vi "dfd_Validate Multirate Filter.vi"(8 "error in (no error)":errorcluster, 9 "skip FXP? (T)":bool=TRUE, 10 "preferred structure":enum16{"CIC", "FIR", "IIR", "Lattice"}(ring), 11 "multirate filter in":T1={"mMRate_Structure"=enum."CIC", "mMRate_Mode"=0, "mMRate_Factor"=1, "mMRate_FIRParams"={"mMRate_FIR_H"=[], "mMRate_FIR_IsNyquist?"=FALSE, "mMRate_FIR_IsSymmetric?"=FALSE}, "mMRate_CICParams"={"mMRate_CIC_#Stage"=2, "mMRate_CIC_Lag"=1, "mMRate_CIC_Type"=enum."Lowpass"}, "mMRate_Order"=1, "mMRate_Version"="1.0", "mMRate_Comments"="1.0", "mMRate_RationalFactor"={"mMRate_L"=-1, "mMRate_M"=-1}, "mMRate_Fs"=0.0, "mMRate_Quantized?"=FALSE, "mMRate_QFilterGain"=1.0, "mMRate_CoefWl"=16, "mMRate_Scaling"={"mMRate_ScaleByPowerOf2?"=FALSE, "mMRate_ScaleType"=enum."Time Domain 1-Norm"}, "mMRate_InputWl"=0, "mMRate_OutputWl"=0, "mMRate_OutputMode"=enum."Nearest", "mMRate_MultMode"=enum."Full", "mMRate_BitPruning"=FALSE, "mMRate_GainWl"=16, "mMRate_OutputFwl"=0, "mMRate_SumIwl"=0, "mMRate_InputIwl "=16, "mMRate_SumWl"=32, "mMRate_CoefIwl"=0} {"mMRate_SumWl" min=1 max=32 step=1; "mMRate_InputIwl" min=1 max=32 step=1; "mMRate_GainWl" min=1 max=32 step=1; "mMRate_OutputWl" min=1 max=32 step=1; "mMRate_InputWl" min=1 max=32 step=1; "mMRate_CoefWl" min=1 max=32 step=1; "mMRate_Mode" items=["Default"=-1, "No Rate Change"=0, "Interpolation"=1, "Decimation"=2, "Interpolated"=3, "Rational"=4]}) -> (0 "error out":errorcluster, 1 "is Valid FXP?":bool, 2 "is Valid FLP?":bool, 3 "multirate filter out":T1={"mMRate_Structure"=enum."CIC", "mMRate_Mode"=0, "mMRate_Factor"=1, "mMRate_FIRParams"={"mMRate_FIR_H"=[], "mMRate_FIR_IsNyquist?"=FALSE, "mMRate_FIR_IsSymmetric?"=FALSE}, "mMRate_CICParams"={"mMRate_CIC_#Stage"=2, "mMRate_CIC_Lag"=1, "mMRate_CIC_Type"=enum."Lowpass"}, "mMRate_Order"=1, "mMRate_Version"="1.0", "mMRate_Comments"="1.0", "mMRate_RationalFactor"={"mMRate_L"=-1, "mMRate_M"=-1}, "mMRate_Fs"=0.0, "mMRate_Quantized?"=FALSE, "mMRate_QFilterGain"=1.0, "mMRate_CoefWl"=16, "mMRate_Scaling"={"mMRate_ScaleByPowerOf2?"=FALSE, "mMRate_ScaleType"=enum."Time Domain 1-Norm"}, "mMRate_InputWl"=0, "mMRate_OutputWl"=0, "mMRate_OutputMode"=enum."Nearest", "mMRate_MultMode"=enum."Full", "mMRate_BitPruning"=FALSE, "mMRate_GainWl"=16, "mMRate_OutputFwl"=0, "mMRate_SumIwl"=0, "mMRate_InputIwl "=16, "mMRate_SumWl"=32, "mMRate_CoefIwl"=0} {"mMRate_SumWl" min=1 max=32 step=1; "mMRate_InputIwl" min=1 max=32 step=1; "mMRate_GainWl" min=1 max=32 step=1; "mMRate_OutputWl" min=1 max=32 step=1; "mMRate_InputWl" min=1 max=32 step=1; "mMRate_CoefWl" min=1 max=32 step=1; "mMRate_Mode" items=["Default"=-1, "No Rate Change"=0, "Interpolation"=1, "Decimation"=2, "Interpolated"=3, "Rational"=4]})   [LabVIEW 2017, in "NI_DigFilterLicensed.lvlib"]
uses:
  <vilib>/addons/Digital Filter Design/NI_DigFilterLicensed.lvlib
  <vilib>/addons/Digital Filter Design/_Objects.llb/DFD Multirate Filter Obj.ctl
  <vilib>/addons/Digital Filter Design/_Objects.llb/DFD Multirate Mode.ctl
  <vilib>/addons/Digital Filter Design/_Objects.llb/DFD Coef Norm Type.ctl
  <vilib>/addons/Digital Filter Design/_Objects.llb/DFD Round-off Mode.ctl
  <vilib>/addons/Digital Filter Design/_Objects.llb/DFD FXP MRate Multiply Mode.ctl
  <vilib>/addons/Digital Filter Design/_Objects.llb/DFD Multirate Rational Factor.ctl
  <vilib>/addons/Digital Filter Design/_Misc.llb/dfd_Error Handlers (Single).vi
  <vilib>/addons/Digital Filter Design/_Misc.llb/dfd_X Equal Y (Scalar).vi
  <vilib>/addons/Digital Filter Design/NI_DigFilter_FXP.lvlib
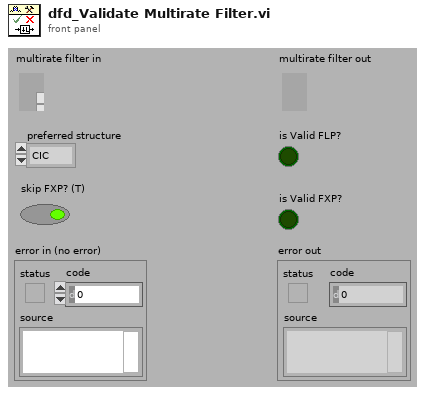
[diagram p1: front panel]
types:
  T1 = typedef "NI_DigFilterLicensed.lvlib/DFD Multirate Filter Obj.ctl" = cluster{"mMRate_Structure":enum16{"CIC", "FIR", "IIR", "Lattice"}, "mMRate_Mode":T2, "mMRate_Factor":i32, "mMRate_FIRParams":cluster{"mMRate_FIR_H":dbl[], "mMRate_FIR_IsNyquist?":bool, "mMRate_FIR_IsSymmetric?":bool}, "mMRate_CICParams":cluster{"mMRate_CIC_#Stage":i32, "mMRate_CIC_Lag":i32, "mMRate_CIC_Type":enum16{"Lowpass", "Highpass"}}, "mMRate_Order":i32, "mMRate_Version":string, "mMRate_Comments":string, "mMRate_RationalFactor":cluster{"mMRate_L":i32, "mMRate_M":i32}, "mMRate_Fs":dbl, "mMRate_Quantized?":bool, "mMRate_QFilterGain":dbl, "mMRate_CoefWl":i16, "mMRate_Scaling":cluster{"mMRate_ScaleByPowerOf2?":bool, "mMRate_ScaleType":T3}, "mMRate_InputWl":i16, "mMRate_OutputWl":i16, "mMRate_OutputMode":T4, "mMRate_MultMode":T5, "mMRate_BitPruning":bool, "mMRate_GainWl":i16, "mMRate_OutputFwl":i16, "mMRate_SumIwl":i16, "mMRate_InputIwl ":i16, "mMRate_SumWl":i16, "mMRate_CoefIwl":i16}
  T2 = typedef "NI_DigFilterLicensed.lvlib/DFD Multirate Mode.ctl" = i16
  T3 = typedef "NI_DigFilterLicensed.lvlib/DFD Coef Norm Type.ctl" = enum16{"No Norm", "Time Domain 1-Norm", "Time Domain 2-Norm", "Time Domain Inf-Norm"}
  T4 = typedef "NI_DigFilterLicensed.lvlib/DFD Round-off Mode.ctl" = enum16{"Nearest", "Truncation"}
  T5 = typedef "NI_DigFilterLicensed.lvlib/DFD FXP MRate Multiply Mode.ctl" = enum16{"Truncated", "Full"}
  T6 = typedef "NI_DigFilterLicensed.lvlib/DFD Multirate Rational Factor.ctl" = cluster{"L":i32, "M":i32}
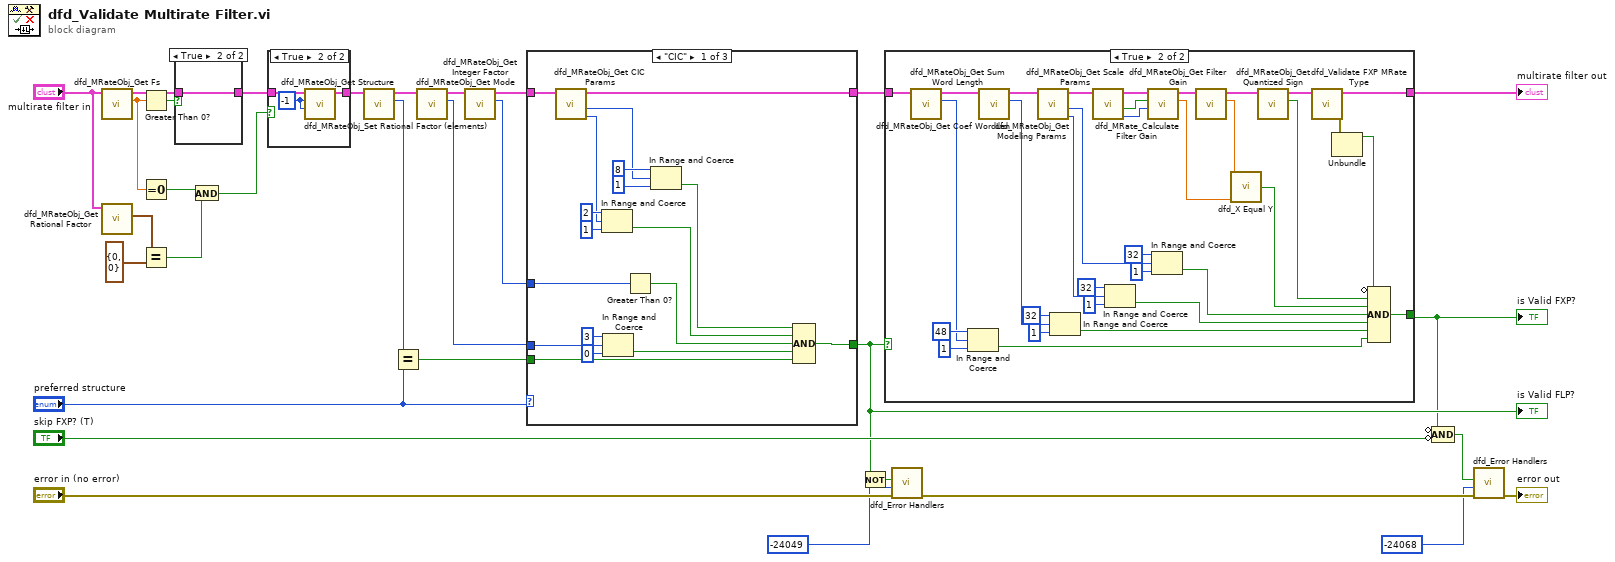
[diagram p0: block diagram]
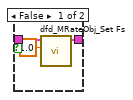
[diagram p3: hidden frame]
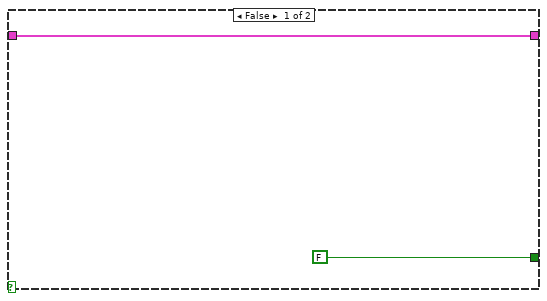
[diagram p4: hidden frame]
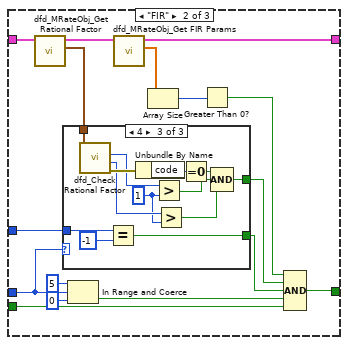
[diagram p5: hidden frame]
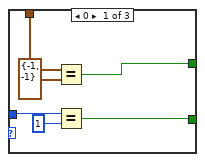
[diagram p6: hidden frame]
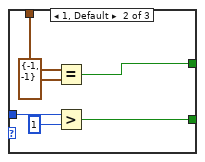
[diagram p7: hidden frame]
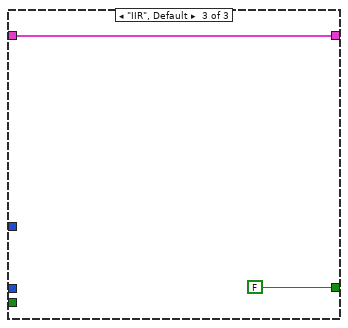
[diagram p8: hidden frame]
diagram:
  n1 = call <vilib>:"dfd_MRateObj_Get Fs.vi"("multirate filter in"="multirate filter in") -> ("fs"=w7:dbl, "dup multirate filter"=w10:T1)  [unwired: 9 out]
  n2 = call <vilib>:"dfd_MRateObj_Get Rational Factor.vi"("multirate filter in"="multirate filter in") -> ("rational factor"=w9:T6)  [unwired: 10 out]
  n3 = Greater Than 0?(x=w7) -> (x > 0?=w11:bool)
  n4 = Equal To 0?(x=w7) -> (x = 0?=w5:bool)
  n5 = Equal?(x=w9, y=T6 {"L"=0, "M"=0}) -> (x = y?=w4:bool)
  n6 = case shown="True" w11 {
    tunnel: w10 -> [w34 w35]
    tunnel: [w33 w35] -> w2
    frame False {
      n7 = call <vilib>:"dfd_MRateObj_Set Fs.vi"("fs"=1.0, "multirate filter in"=w34) -> ("dup multirate filter"=w33:T1)  [unwired: 9 out]
    }
    frame True {
    }
  }
  n8 = And(x=w5, y=w4) -> (x .and. y?=w3:bool)
  n9 = case shown="True" w3 {
    tunnel: w2 -> [w36 w39]
    tunnel: [w36 w38] -> w1
    frame False {
    }
    frame True {
      w37 = -1 ("L")
      n10 = call <vilib>:"dfd_MRateObj_Set Rational Factor (elements).vi"("M"=w37, "L"=w37, "multirate filter in"=w39) -> ("multirate filter out"=w38:T1)  [unwired: 8 out]
    }
  }
  n11 = call <vilib>:"dfd_MRateObj_Get Structure.vi"("multirate filter in"=w1) -> ("structure"=w21:enum16{"CIC", "FIR", "IIR", "Lattice"}, "dup multirate filter"=w23:T1)  [unwired: 9 out]
  n12 = Equal?(x=w21, y="preferred structure") -> (x = y?=w19:bool)
  n13 = call <vilib>:"dfd_MRateObj_Get Mode.vi"("multirate filter in"=w23) -> ("mode"=w18:T2, "dup multirate filter"=w22:T1)  [unwired: 9 out]
  n14 = call <vilib>:"dfd_MRateObj_Get Integer Factor.vi"("multirate filter in"=w22) -> ("factor"=w17:i32, "dup multirate filter"=w12:T1)  [unwired: 9 out]
  n15 = case shown="\"CIC\"" "preferred structure" {
    tunnel: [w46 w72 FALSE] -> w16
    tunnel: w19 -> [w52 w69 _]
    tunnel: w18 -> [w57 w67 _]
    tunnel: w17 -> [w54 w66 _]
    tunnel: w12 -> [w53 w68 w99]
    tunnel: [w40 w62 w99] -> w15
    frame "CIC" {
      n16 = call <vilib>:"dfd_MRateObj_Get CIC Params.vi"("multirate filter in"=w53) -> ("lag"=w48:i32, "# stages"=w41:i32, "dup multirate filter"=w40:T1)  [unwired: 8 out]
      n17 = In Range and Coerce(upper limit=2, x=w48, lower limit=1) -> (In Range?=w47:bool)  [unwired: 1 out]
      n18 = In Range and Coerce(upper limit=i16 3, x=w57, lower limit=i16 0) -> (In Range?=w51:bool)  [unwired: 1 out]
      n19 = Greater Than 0?(x=w54) -> (x > 0?=w45:bool)
      n20 = In Range and Coerce(upper limit=8, x=w41, lower limit=1) -> (In Range?=w42:bool)  [unwired: 1 out]
      n21 = Compound Arithmetic op=AND(w42, w47, w45, w51, w52) -> (w46:bool)
    }
    frame "FIR" {
      n22 = call <vilib>:"dfd_MRateObj_Get Rational Factor.vi"("multirate filter in"=w68) -> ("rational factor"=w65:T6, "dup multirate filter"=w64:T1)  [unwired: 9 out]
      n23 = case shown="4" w67 {
        tunnel: w66 -> [w75 w81 w98]
        tunnel: w65 -> [w79 w85 w94]
        tunnel: [w76 w82 w93] -> w60
        tunnel: [w77 w83 w89] -> w59
        frame 0 {
          n24 = Equal?(x=w79, y=T6 {"L"=-1, "M"=-1}) -> (x = y?=w77:bool)
          n25 = Equal?(x=w75, y=1) -> (x = y?=w76:bool)
        }
        frame 1, Default {
          n26 = Equal?(x=w85, y=T6 {"L"=-1, "M"=-1}) -> (x = y?=w83:bool)
          n27 = Greater?(x=w81, y=1) -> (0:w82:bool)
        }
        frame 4 {
          w90 = 1 ("y")
          n28 = call <vilib>:"dfd_Check Rational Factor.vi"("rational factor in"=w94) -> ("error out"=w95:errorcluster, "M"=w91:i32, "L"=w92:i32)  [unwired: 1 in, 7 out]
          n29 = Equal?(x=w98, y=-1) -> (x = y?=w93:bool)
          n30 = Unbundle By Name(w95) -> ("code"=w96:i32)
          n31 = Greater?(x=w92, y=w90) -> (0:w86:bool)
          n32 = Greater?(x=w91, y=w90) -> (0:w88:bool)
          n33 = Equal To 0?(x=w96) -> (x = 0?=w87:bool)
          n34 = Compound Arithmetic op=AND(w87, w86, w88) -> (w89:bool)
        }
      }
      n35 = In Range and Coerce(upper limit=i16 5, x=w67, lower limit=i16 0) -> (In Range?=w61:bool)  [unwired: 1 out]
      n36 = call <vilib>:"dfd_MRateObj_Get FIR Params.vi"("multirate filter in"=w64) -> ("h(n)"=w63:dbl[], "dup multirate filter"=w62:T1)  [unwired: 9 out]
      n37 = Array Size(array=w63) -> (size(s)=w73:i32)
      n38 = Greater Than 0?(x=w73) -> (x > 0?=w58:bool)
      n39 = Compound Arithmetic op=AND(w58, w59, w60, w61, w69) -> (w72:bool)
    }
    frame "IIR", Default {
    }
  }
  "is Valid FLP?" <- w16
  n40 = Not(x=w16) -> (.not. x?=w29:bool)
  n41 = case shown="True" w16 {
    tunnel: w15 -> [w102 w108]
    tunnel: [w102 w111] -> w14
    tunnel: [FALSE w113] -> w13
    frame False {
    }
    frame True {
      n42 = call <vilib>:"dfd_MRateObj_Get Sum Word Length.vi"("multirate filter in"=w108) -> ("SumWl"=w104:i16, "multirate filter out"=w107:T1)  [unwired: 9 out]
      n43 = In Range and Coerce(upper limit=i16 48, x=w104, lower limit=i16 1) -> (In Range?=w103:bool)  [unwired: 1 out]
      n44 = call <vilib>:"dfd_MRateObj_Get Coef WordLen.vi"("multirate filter in"=w107) -> ("coef wl"=w131:i16, "dup multirate filter"=w136:T1)  [unwired: 9 out]
      n45 = call <vilib>:"dfd_MRateObj_Get Modeling Params.vi"("multirate filter in"=w136) -> ("output wl"=w124:i16, "input wl"=w123:i16, "dup multirate filter"=w119:T1)  [unwired: 8 out]
      n46 = In Range and Coerce(upper limit=i16 32, x=w131, lower limit=i16 1) -> (In Range?=w122:bool)  [unwired: 1 out]
      n47 = call <vilib>:"dfd_MRateObj_Get Scale Params.vi"("multirate filter in"=w119) -> ("scale type"=w133:T3, "scale by Power of 2?"=w134:bool, "dup multirate filter"=w135:T1)  [unwired: 8 out]
      n48 = In Range and Coerce(upper limit=i16 32, x=w124, lower limit=i16 1) -> (In Range?=w121:bool)  [unwired: 1 out]
      n49 = call <vilib>:"dfd_MRate_Calculate Filter Gain.vi"("scale type"=w133, "scale by Power of 2?"=w134, "multirate filter in"=w135) -> ("scaled gain"=w115:dbl, "dup multirate filter"=w132:T1)  [unwired: 7 out]
      n50 = In Range and Coerce(upper limit=i16 32, x=w123, lower limit=i16 1) -> (In Range?=w120:bool)  [unwired: 1 out]
      n51 = call <vilib>:"dfd_MRateObj_Get Filter Gain.vi"("multirate filter in"=w132) -> ("gain"=w116:dbl, "dup multirate filter"=w118:T1)  [unwired: 9 out]
      n52 = call-poly <vilib>:"dfd_X Equal Y.vi"("x"=w116, "y"=w115) -> ("x = y?"=w114:bool)  [unwired: 1 in, 4 out]
      n53 = call <vilib>:"dfd_MRateObj_Get Quantized Sign.vi"("multirate filter in"=w118) -> ("is Quantized?"=w117:bool, "dup multirate filter"=w112:T1)  [unwired: 9 out]
      n54 = call <vilib>:"dfd_Validate FXP MRate Type.vi"("multirate filter in"=w112) -> ("error out"=w110:errorcluster, "dup multirate filter"=w111:T1)  [unwired: 1 in, 8 out]
      n55 = Unbundle(w110) -> ("status"=w109:bool)  [unwired: 2 out]
      n56 = Compound Arithmetic op=AND(invert w109, w117, w114, w120, w121, w122, w103) -> (w113:bool)
    }
  }
  "multirate filter out" <- w14
  "is Valid FXP?" <- w13
  n57 = call-poly <vilib>:"dfd_Error Handlers.vi"("error in (no error)"="error in (no error)", "error code"=-24049 ("ERR_INVALID_MULTIRATE_FILTER"), "condition failed?"=w29) -> ("error out"=w27:errorcluster)  [unwired: 8 out]
  n58 = Compound Arithmetic op=AND(invert w13, invert "skip FXP? (T)") -> (w25:bool)
  n59 = call-poly <vilib>:"dfd_Error Handlers.vi"("error in (no error)"=w27, "error code"=-24068 ("ERR_INVALID_FXP_MRATE"), "condition failed?"=w25) -> ("error out"=→"error out":errorcluster)  [unwired: 8 out]
